vi "WriteTempSensorParam332.vi"(3 "Error in":errorcluster, 5 "SensorPar":T1={"TableTC"=1, "TableConv"=1, "Compensation"=1, "Type"=9} caption="Paramètre de configuration d'entrée" {"Compensation" items=["Off", "On"]; "TableConv" max=60 step=1; "Type" items=["Silicon Diode", "GaAlAs Diode", "Platinum 100 (250 Ohms)", "Platinum 100 (500 Ohms)", "Platinum 1000 Ohms", "NTC RTD 75mV 7.5 KOhms", "Thermocouple 25mV", "Thermocouple 50mV", "NTC RTD 75mV 75 Ohms", "NTC RTD 75mV 750 Ohms", "NTC RTD 75mV 7.5 KOhms", "NTC RTD 75mV 75 KOhms", "NTC RTD 75mV Auto"]; "TableTC" max=41 step=1}, 6 "Nom":string) -> (0 "Error out":errorcluster, 1 "SavedOK":bool, 2 "Configurations":string[](array[string]))   [LabVIEW 2010]
doc: "Ce VI sauvegarde les modèles de configuration créer à l'intérieur du fichier de modèles."
uses:
  InConfigPar332.ctl
  <vilib>/Utility/config.llb/Write Key (I32).vi
  <vilib>/Utility/config.llb/NI_LVConfig.lvlib
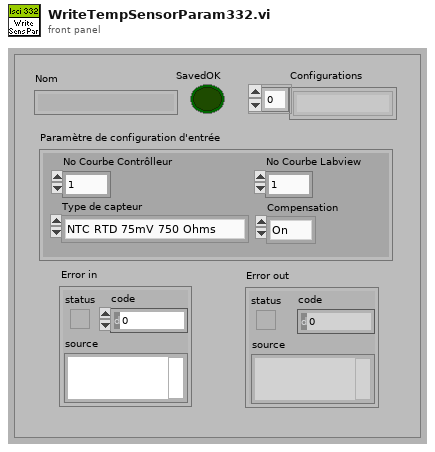
[diagram p1: front panel]
types:
  T1 = typedef "InConfigPar332.ctl" = cluster{"TableTC":u16, "TableConv":u16, "Compensation":u16, "Type":u16}
  T2 = typedef "NI_LVConfig.lvlib/Config Data RefNum.ctl" = refnum<k1>
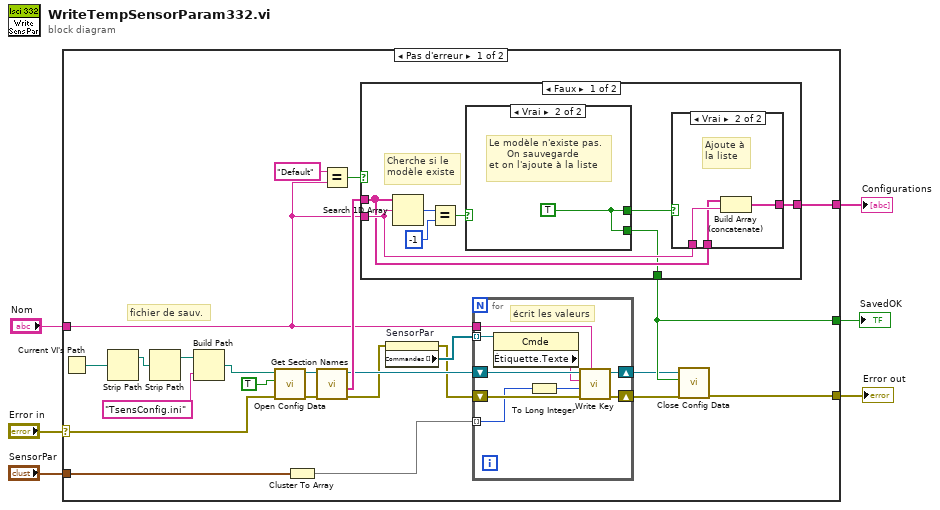
[diagram p0: block diagram]
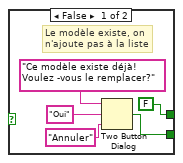
[diagram p3: hidden frame]
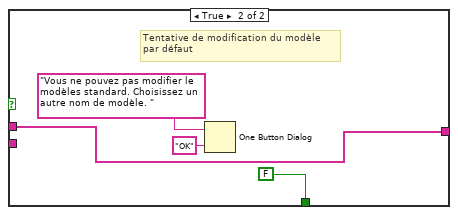
[diagram p4: hidden frame]
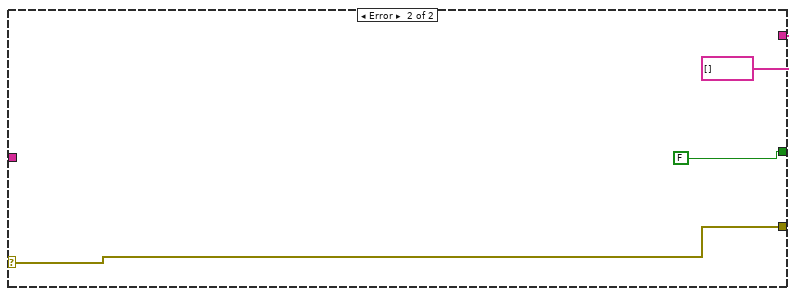
[diagram p5: hidden frame]
diagram:
  n1 = case shown="Pas d'erreur" "Error in" {
    selector: "Error in" -> [w28 w64]
    tunnel: "Nom" -> [w20 _]
    tunnel: [w29 w64] -> w5
    tunnel: [w21 FALSE ("T button?")] -> w3
    tunnel: [w22 string[] [] ("section names")] -> w2
    tunnel: "SensorPar" -> [w15 _]
    frame No Error {
      # "fichier de sauv."
      n2 = Current VI's Path() -> (path=w11:path)
      n3 = Strip Path(path=w11) -> (stripped path=w9:path)  [unwired: 1 out]
      n4 = Strip Path(path=w9) -> (stripped path=w8:path)  [unwired: 1 out]
      n5 = Build Path(base path=w8, name or relative path="TsensConfig.ini") -> (appended path=w7:path)
      n6 = call <vilib>:"Open Config Data.vi"("error in (no error)"=w28, "create file if necessary (T)"=TRUE ("create file if necessary? (T)"), "configuration file path"=w7) -> ("error out"=w27:errorcluster, "refnum"=w26:T2)  [unwired: 6 in, 1 out]
      n7 = Cluster To Array(cluster=w15) -> (array=w14:u16[])
      n8 = call <vilib>:"Get Section Names.vi"("error in (no error)"=w27, "refnum"=w26) -> ("error out"=w13:errorcluster, "section names"=w23:string[], "refnum out"=w18:T2)  [unwired: 7 in]
      n9 = Equal?(x="Default", y=w20) -> (x = y?=w24:bool)
      n10 = case shown="Faux" w24 {
        tunnel: [w41 FALSE] -> w21
        tunnel: w23 -> [w43 w58]
        tunnel: w20 -> [w44 _]
        tunnel: [w42 w58] -> w22
        frame False {
          # "Cherche si le\nmodèle existe"
          n11 = Search 1D Array(1D array=w43, element=w44) -> (index of element=w47:i32)  [unwired: 1 in]
          n12 = Equal?(x=w47, y=-1) -> (x = y?=w45:bool)
          n13 = case shown="Vrai" w45 {
            tunnel: [FALSE w57] -> w40
            tunnel: [w53 w57] -> w41
            frame False {
              # "Le modèle existe, on n'ajoute pas à la liste"
              n14 = Two Button Dialog(message="Ce modèle existe déjà! Voulez -vous le remplacer?", 1:"Annuler" ("F button name (\"Cancel\")"), 2:"Oui" ("T button name (\"OK\")")) -> (T button?=w53:bool)
            }
            frame True {
              w57 = TRUE
              # "Le modèle n'existe pas.\n      On sauvegarde\net on l'ajoute à la liste"
            }
          }
          n15 = case shown="Vrai" w40 {
            tunnel: w44 -> [_ w51]
            tunnel: w43 -> [w48 w50]
            tunnel: [w48 w49] -> w42
            frame False {
            }
            frame True {
              # "Ajoute à\nla liste"
              n16 = Build Array (concatenate)(w50, w51) -> (w49:string[])
            }
          }
        }
        frame True {
          # "Tentative de modification du modèle\npar défaut"
          n17 = One Button Dialog(message="Vous ne pouvez pas modifier le modèles standard. Choisissez un autre nom de modèle. ", button name ("OK")="OK") -> ()  [unwired: 1 out]
        }
      }
      n18 = property on="SensorPar" class="Clust (strict)"(error in=w13) -> (error out=w12:errorcluster, "Commandes []"=w16:refnum<vi>[])  [unwired: 1 in, 1 out]
      n19 = for {
        tunnel: w20 -> [w39]
        shift-right: [w38] -> w19
        shift-left: w18 -> [w37]
        shift-right: [w36] -> w17
        shift-left: w12 -> [w34]
        tunnel: w16 -> [w33] mode=indexing
        tunnel: w14 -> [w32] mode=indexing
        # "écrit les valeurs"
        n20 = property class="Cmde"(reference=w33) -> ("Étiquette.Texte"=w35:string)  [unwired: 1 in, 2 out]
        n21 = To Long Integer(number=w32) -> (32bit integer=w31:i32)
        n22 = call-poly <vilib>:"Write Key.vi"("section"=w39, "error in (no error)"=w34, "value"=w31, "key"=w35, "refnum"=w37) -> ("error out"=w36:errorcluster, "refnum out"=w38:T2)  [unwired: 4 in, 1 out]
      }
      n23 = call <vilib>:"Close Config Data.vi"("error in (no error)"=w17, "write file if changed (T)"=w21, "refnum"=w19) -> ("error out"=w29:errorcluster)  [unwired: 7 in, 1 out]
    }
    frame Error {
    }
  }
  "Error out" <- w5
  "SavedOK" <- w3
  "Configurations" <- w2
